vi "Line.vi"(4 "Properties":T1={"Line"={"Style"=enum."Automatic", "Color"=2147483647, "Width"=nan}, "Marker"={"Style"=enum."Automatic", "Color"=2147483647, "Size"=nan}, "Display"={"Alpha"=nan, "Z Order"=nan}} {"Marker"."Color" items=["Automatic"=2147483647, "Black"=0, "White"=16777215, "Red"=16711680, "Green"=2263842, "Blue"=255, "Cyan"=65535, "Magenta"=16711935, "Yellow"=16776960]; "Line"."Color" items=["Automatic"=2147483647, "Black"=0, "White"=16777215, "Red"=16711680, "Green"=2263842, "Blue"=255, "Cyan"=65535, "Magenta"=16711935, "Yellow"=16776960]}, 6 "Legend Title":string, 8 "error in (no error)":errorcluster, 9 "Y Data":dbl[](array[numeric]), 10 "X Data":dbl[](array[numeric]), 11 "Plot ID":T8 format="%x") -> (0 "error out":errorcluster, 3 "Plot ID out":T8 format="%x")   [LabVIEW 2013, in "Advanced Plotting Toolkit.lvlib"]
doc: "Make a line plot, from X and Y data. By default, only the line is shown; markers are not."
uses:
  Advanced Plotting Toolkit.lvlib
  typedefs/PlotID.ctl
  LineProperties.ctl
  properties/Line.ctl
  properties/Line_Style.ctl
  typedefs/PlotColor.ctl
  properties/Marker.ctl
  properties/Marker_Style.ctl
  properties/Display.ctl
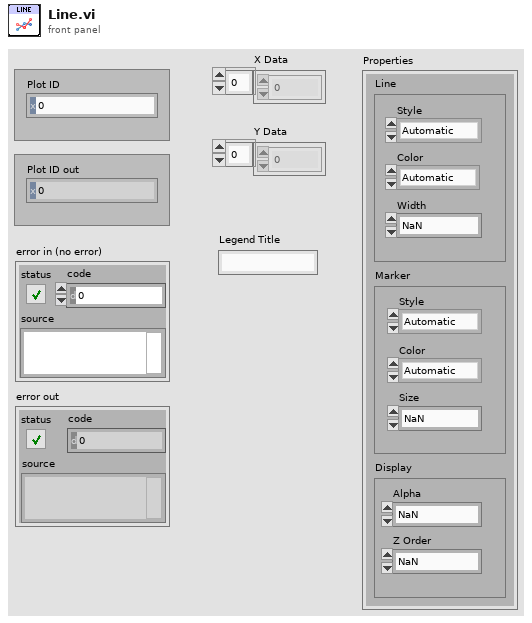
[diagram p1: front panel]
types:
  T1 = typedef "Advanced Plotting Toolkit.lvlib/LineProperties.ctl" = cluster{"Line":T2, "Marker":T5, "Display":T7}
  T2 = typedef "Advanced Plotting Toolkit.lvlib/Line.ctl" = cluster{"Style":T3, "Color":T4, "Width":sgl}
  T3 = typedef "Advanced Plotting Toolkit.lvlib/Line_Style.ctl" = enum16{"Automatic", "Solid", "Dashed", "Dotted", "Dash-dot", "Invisible"}
  T4 = typedef "Advanced Plotting Toolkit.lvlib/PlotColor.ctl" = u32
  T5 = typedef "Advanced Plotting Toolkit.lvlib/Marker.ctl" = cluster{"Style":T6, "Color":T4, "Size":dbl}
  T6 = typedef "Advanced Plotting Toolkit.lvlib/Marker_Style.ctl" = enum16{"Automatic", "Circle", "Square", "Triangle", "Diamond", "Star", "Invisible"}
  T7 = typedef "Advanced Plotting Toolkit.lvlib/Display.ctl" = cluster{"Alpha":dbl, "Z Order":dbl}
  T8 = typedef "Advanced Plotting Toolkit.lvlib/PlotID.ctl" = i32
  T9 = typedef "Advanced Plotting Toolkit.lvlib/KeyValue.ctl" = cluster{"Key":string, "Value":string}
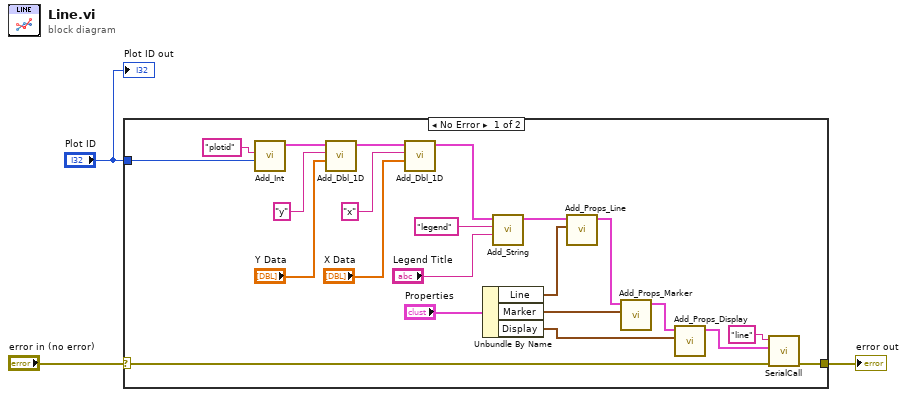
[diagram p0: block diagram]
diagram:
  n1 = case shown="No Error" "error in (no error)" {
    selector: "error in (no error)" -> [w16 w26]
    tunnel: [w23 w26] -> w3
    tunnel: "Plot ID" -> [w13 _]
    frame No Error {
      n2 = call "Add_Int.vi"("Value"=w13, "Key"="plotid" ("Keyword")) -> ("Keyword Array Out"=w22:T9[])  [unwired: 9 in]
      n3 = call "Add_Dbl_1D.vi"("Value"="Y Data", "Key"="y", "Keyword Array"=w22) -> ("Keyword Array Out"=w20:T9[])  [unwired: 8 in]
      n4 = call "Add_Dbl_1D.vi"("Value"="X Data", "Key"="x", "Keyword Array"=w20) -> ("Keyword Array Out"=w7:T9[])  [unwired: 8 in]
      n5 = Unbundle By Name("Properties") -> ("Line"=w12:T2, "Marker"=w11:T5, "Display"=w9:T7)
      n6 = call "Add_String.vi"("Value"="Legend Title", "Key"="legend", "Keyword Array"=w7) -> ("Keyword Array Out"=w6:T9[])  [unwired: 8 in]
      n7 = call "Add_Props_Line.vi"("Line"=w12, "Keyword Array"=w6) -> ("Keyword Array Out"=w17:T9[])  [unwired: 9 in]
      n8 = call "Add_Props_Marker.vi"("Marker"=w11, "Keyword Array"=w17) -> ("Keyword Array Out"=w10:T9[])  [unwired: 9 in]
      n9 = call "Add_Props_Display.vi"("Display"=w9, "Keyword Array"=w10) -> ("Keyword Array Out"=w8:T9[])  [unwired: 9 in]
      n10 = call "SerialCall.vi"("error in (no error)"=w16, "data"=w8, "Resource"="line") -> ("error out"=w23:errorcluster)  [unwired: 7 in, 1 out]
    }
    frame Error {
    }
  }
  "error out" <- w3
  "Plot ID out" <- "Plot ID"
